vi "SiosIfmSetFilterNotchFrequency.vi"(1 "FilterStage1NotchCoeff":dbl, 2 "channel":i32, 3 "DeviceNumber":i32) -> (0 "success":i32)   [LabVIEW 2009]
uses:
  siosifm.dll
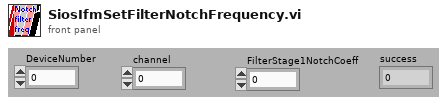
[diagram p1: front panel]
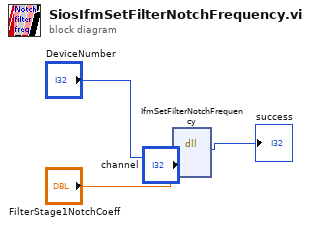
[diagram p0: block diagram]
diagram:
  n1 = dll-call lib="D:/Support/Labview/RE-10/SIOS_IfmDLL/siosifm.dll" fn="IfmSetFilterNotchFrequency"("devNumber"="DeviceNumber", "channel"="channel", "frequency"="FilterStage1NotchCoeff") -> (→"success":i32)  [unwired: 6 in, 2 out]
